vi "Initialize Library.vi"   [LabVIEW 2021]
uses:
  <userlib>/SciSDK/SciSDK_Labview.lvlib
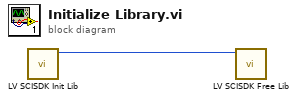
[diagram p0: block diagram]
diagram:
  n1 = call <userlib>:"LV SCISDK Init Lib.vi"() -> ("function return"=w1:u64)  [unwired: 11 in]
  n2 = call <userlib>:"LV SCISDK Free Lib.vi"("handle"=w1) -> ()  [unwired: 9 in, 2 out]
